vi "stop.vi"(8 "error in (no error)":errorcluster, 10 "stop?":bool, 11 "CQT_DDS in":refnum<class "CQT_DDS.lvclass">) -> (0 "error out":errorcluster, 2 "hasStopped":bool, 3 "CQT_DDS out":refnum<class "CQT_DDS.lvclass">)   [LabVIEW 2011, in "CQT_DDS.lvclass"]
uses:
  CQT_DDS.lvclass
  CQT_DDS.lvclass/CQT_DDS.ctl
  C:/Program Files/National Instruments/LabVIEW 2011/instr.lib/CQT_DDS/DDSLibrary/20111109/CQTAD9958.dll
  Program Files/National Instruments/LabVIEW 2011/instr.lib/CQT_DDS/DDSLibrary/20111109/CQTAD9958.dll
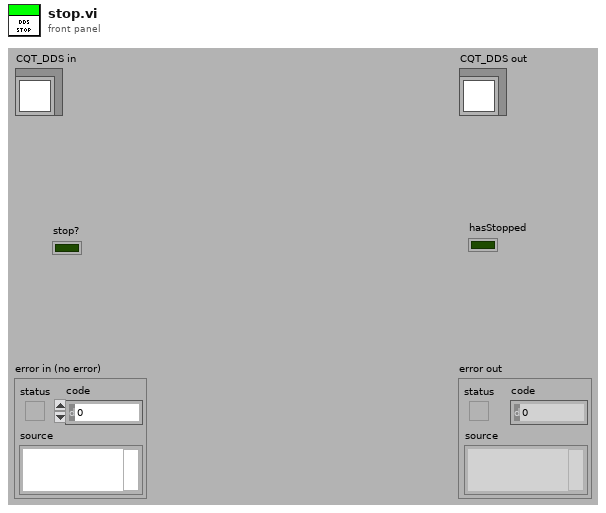
[diagram p1: front panel]
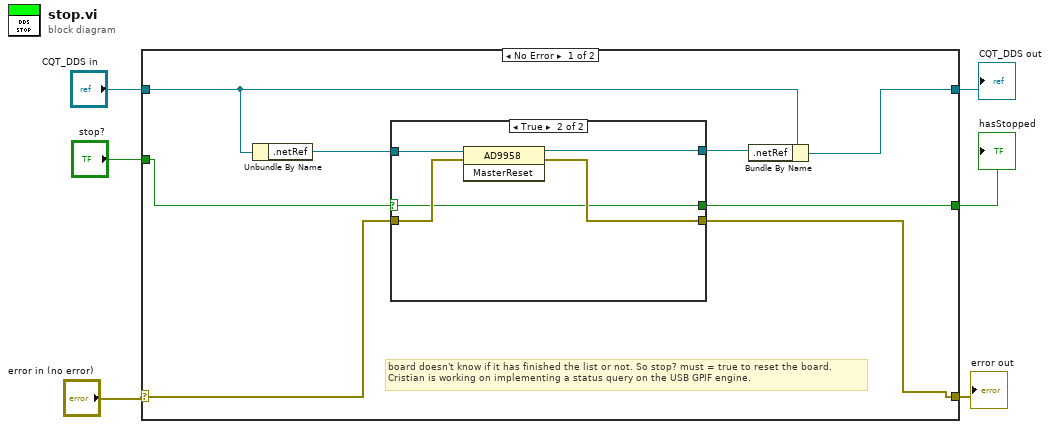
[diagram p0: block diagram]
diagram:
  n1 = case shown="No Error" "error in (no error)" {
    selector: "error in (no error)" -> [w12 w24]
    tunnel: "CQT_DDS in" -> [w10 w23]
    tunnel: [w9 w23] -> w4
    tunnel: [w11 w24] -> w3
    tunnel: "stop?" -> [w13 _]
    tunnel: [w7 _] -> w1
    frame No Error {
      # "board doesn't know if it has finished the list or not. So stop? must = true to reset the board.\nCristian is working on implementing a status query on the USB GPIF engine."
      n2 = Unbundle By Name(w10) -> (".netRef"=w14:refnum<k24>)
      n3 = case shown="True" w13 {
        selector: w13 -> [w15 w18]
        tunnel: w14 -> [w17 w22]
        tunnel: w12 -> [w16 w21]
        tunnel: [w16 w20] -> w11
        tunnel: [w17 w19] -> w8
        tunnel: [w15 w18] -> w7
        frame False {
        }
        frame True {
          n4 = invoke class="AD9958" method="MasterReset"(reference=w22, error in=w21) -> (reference out=w19:refnum<k24>, error out=w20:errorcluster)  [unwired: 1 in, 1 out]
        }
      }
      n5 = Bundle By Name(cluster=w10, ".netRef"=w8) -> (w9:refnum<class "CQT_DDS.lvclass">)
    }
    frame Error {
    }
  }
  "error out" <- w3
  "CQT_DDS out" <- w4
  "hasStopped" <- w1
